vi "rotation_matrix.vi"(0 "Rotation":dbl, 1 "Translation X":dbl, 2 "Translation Y":dbl, 3 "Translation Z":dbl, 4 "Enum":enum16{"x", "y", "z"}(ring)) -> (5 "Real Matrix":T1)   [LabVIEW 2019]
uses:
  <vilib>/Analysis/Matrix/Datatypes/RealMatrix.ctl
  <vilib>/Analysis/Matrix/NI_Matrix.lvlib
panel:
  out "Real Matrix 2":T1
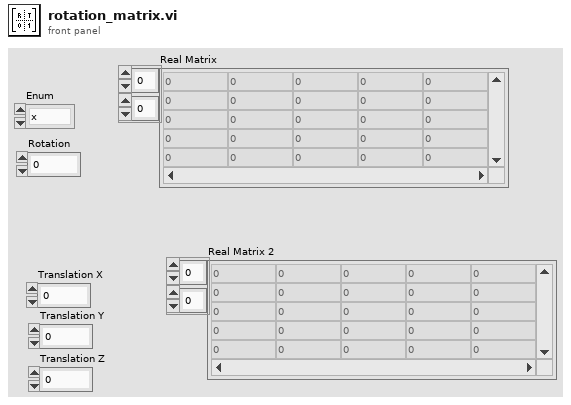
[diagram p1: front panel]
types:
  T1 = typedef "NI_Matrix.lvlib/RealMatrix.ctl" = dbl[][]
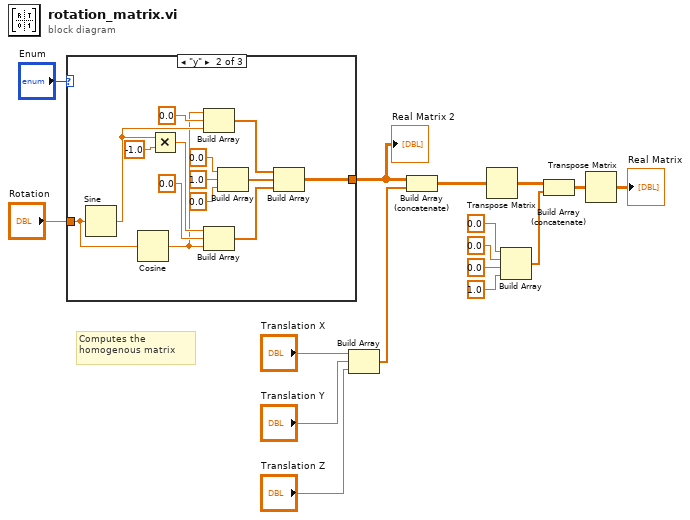
[diagram p0: block diagram]
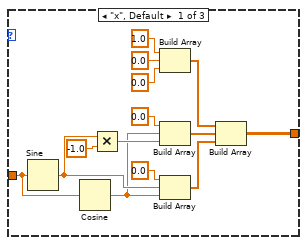
[diagram p2: hidden frame]
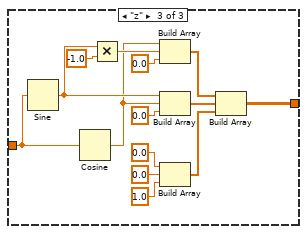
[diagram p3: hidden frame]
diagram:
  # "Computes the homogenous matrix"
  n1 = case shown="\"y\"" "Enum" {
    tunnel: "Rotation" -> [w22 w40 w46]
    tunnel: [w17 w31 w45] -> w1
    frame "x", Default {
      n2 = Sine(x=w22) -> (sin(x)=w19:dbl)
      n3 = Cosine(x=w22) -> (cos(x)=w18:dbl)
      n4 = Multiply(x=w19, y=-1.0) -> (x*y=w21:dbl)
      n5 = Build Array(1.0 ("element"), 0.0 ("element"), 0.0 ("element")) -> (w27:dbl[])
      n6 = Build Array(0.0 ("element"), w18, w21) -> (w26:dbl[])
      n7 = Build Array(0.0 ("element"), w19, w18) -> (w25:dbl[])
      n8 = Build Array(w27, w26, w25) -> (w17:T1)
    }
    frame "y" {
      n9 = Sine(x=w40) -> (sin(x)=w39:dbl)
      n10 = Cosine(x=w40) -> (cos(x)=w32:dbl)
      n11 = Multiply(x=w39, y=-1.0) -> (x*y=w34:dbl)
      n12 = Build Array(w32, 0.0 ("element"), w39) -> (w44:dbl[])
      n13 = Build Array(w34, 0.0 ("element"), w32) -> (w42:dbl[])
      n14 = Build Array(0.0 ("element"), 1.0 ("element"), 0.0 ("element")) -> (w43:dbl[])
      n15 = Build Array(w44, w43, w42) -> (w31:T1)
    }
    frame "z" {
      n16 = Sine(x=w46) -> (sin(x)=w52:dbl)
      n17 = Cosine(x=w46) -> (cos(x)=w51:dbl)
      n18 = Multiply(x=w52, y=-1.0) -> (x*y=w54:dbl)
      n19 = Build Array(w51, w54, 0.0 ("element")) -> (w58:dbl[])
      n20 = Build Array(w52, w51, 0.0 ("element")) -> (w57:dbl[])
      n21 = Build Array(0.0 ("element"), 0.0 ("element"), 1.0 ("element")) -> (w56:dbl[])
      n22 = Build Array(w58, w57, w56) -> (w45:T1)
    }
  }
  "Real Matrix 2" <- w1
  n23 = Build Array("Translation X", "Translation Y", "Translation Z") -> (w14:dbl[])
  n24 = Build Array (concatenate)(w1, w14) -> (w10:T1)
  n25 = Transpose Matrix(1:w10) -> (0:w9:T1)
  n26 = Build Array(0.0 ("element"), 0.0 ("element"), 0.0 ("element"), 1.0 ("element")) -> (w4:dbl[])
  n27 = Build Array (concatenate)(w9, w4) -> (w3:T1)
  n28 = Transpose Matrix(1:w3) -> (0:→"Real Matrix":T1)
